vi "QI_80_ver1.vi"(6 "x_qi in":sgl, 7 "y_qi in":sgl, 9 "arraySize":i32, 10 "Array 2":sgl[](array[numeric]), 11 "Array":sgl[][](array[numeric])) -> (1 "y_qi out":sgl, 2 "x_qi out":sgl, 3 "rdp_profile":sgl[](array[numeric]))   [LabVIEW 2017]
uses:
  C:/Users/user/Documents/Visual Studio 2015/Projects/cudadll/QIdllv1/cudadll.dll
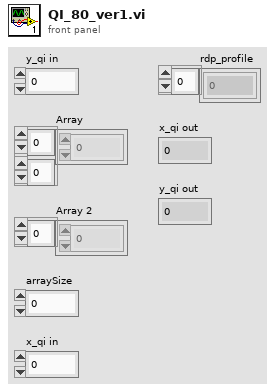
[diagram p1: front panel]
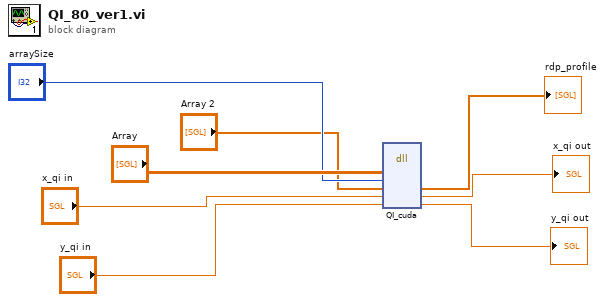
[diagram p0: block diagram]
diagram:
  n1 = dll-call lib="C:/Users/user/Documents/Visual Studio 2015/Projects/cudadll/QIdllv1/cudadll.dll" fn="QI_cuda"("img_mat"="Array", "arraySize"="arraySize", "rdp_profile"="Array 2", "x_qi"="x_qi in", "y_qi"="y_qi in") -> ("rdp_profile"=→"rdp_profile":sgl[], "x_qi"=→"x_qi out":sgl, "y_qi"=→"y_qi out":sgl)  [unwired: 6 in, 2 out]
